vi "cm2nm_index_and_pair_fiducials.vi"(2 "CurrentSessionCollectionOfPoints":T1[](array[typedef]), 4 "ReferenceSessionCollectionOfPoints":T1[](array[typedef]), 5 "IndexCurrentSession_PairingList":i32[](array[numeric]), 6 "ReplacePairedFidName":bool, 7 "ReferenceSessionFiducialIndex":i32[](array[numeric]), 8 "CurrentSessionFiducialIndex":i32[](array[numeric]), 9 "IndexRefrenceSession_PairlingList":i32[](array[numeric])) -> (0 "CurrentSessionOut":T1[](array[typedef])=[{"MetaDataFile"=path "", "X"=-1.1, "Y"=0.0, "Z"=0.0, "Group"=0, "Rotation"=0.0, "Fiducial"=TRUE, "Magnification"=0.0, "Working_Distance"=0.0, "Notes"="", "Location Name/ID"="", "OtherRelatedDataFiles"=[], "Available"=FALSE}, {"MetaDataFile"=path "", "X"=0.0, "Y"=-1.0, "Z"=0.0, "Group"=0, "Rotation"=0.0, "Fiducial"=TRUE, "Magnification"=0.0, "Working_Distance"=0.0, "Notes"="", "Location Name/ID"="", "OtherRelatedDataFiles"=[], "Available"=FALSE}, {"MetaDataFile"=path "", "X"=0.0, "Y"=1.0, "Z"=0.0, "Group"=0, "Rotation"=0.0, "Fiducial"=TRUE, "Magnification"=0.0, "Working_Distance"=0.0, "Notes"="", "Location Name/ID"="", "OtherRelatedDataFiles"=[], "Available"=FALSE}, {"MetaDataFile"=path "", "X"=1.0, "Y"=0.0, "Z"=0.0, "Group"=0, "Rotation"=0.0, "Fiducial"=TRUE, "Magnification"=0.0, "Working_Distance"=0.0, "Notes"="", "Location Name/ID"="", "OtherRelatedDataFiles"=[], "Available"=FALSE}], 1 "PairedFiducialNames":T2(array[cluster]), 3 "PairedFiducials":T3(array[cluster]))   [LabVIEW 2011]
doc: "This Vi extracts the paired coordinates and names and puts into the format that the coordinate transform functions where created. Just book keeping."
uses:
  cm2nm_coordinate_information_v2.ctl
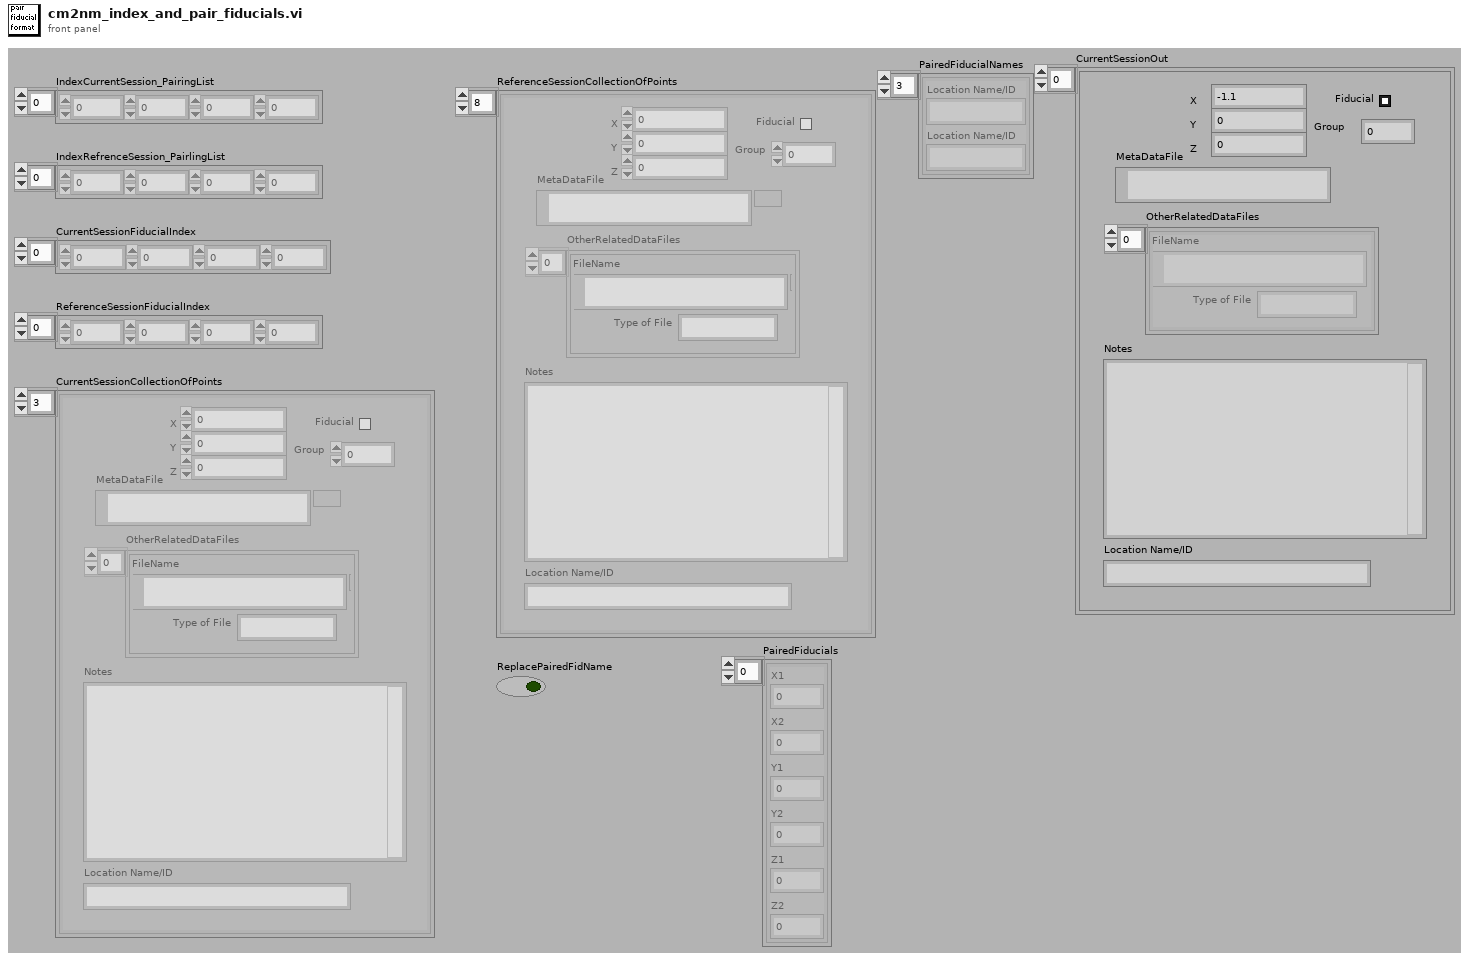
[diagram p1: front panel]
types:
  T1 = typedef "cm2nm_coordinate_information_v2.ctl" = cluster{"MetaDataFile":path, "X":dbl, "Y":dbl, "Z":dbl, "Group":i32, "Rotation":dbl[unit], "Fiducial":bool, "Magnification":dbl, "Working_Distance":dbl, "Notes":string, "Location Name/ID":string, "OtherRelatedDataFiles":cluster{"Type of File":string, "FileName":path}[], "Available":bool}
  T2 = cluster{"Location Name/ID":string, "Location Name/ID":string}[]
  T3 = cluster{"X1":dbl, "X2":dbl, "Y1":dbl, "Y2":dbl, "Z1":dbl, "Z2":dbl}[]
  T4 = cluster{"X1":dbl, "X2":dbl, "Y1":dbl, "Y2":dbl, "Z1":dbl, "Z2":dbl}
  T5 = cluster{"Location Name/ID":string, "Location Name/ID":string}
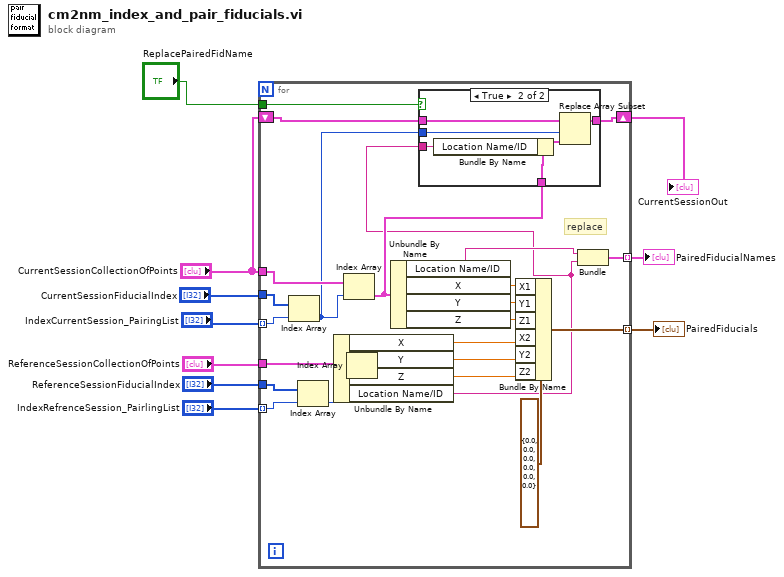
[diagram p0: block diagram]
diagram:
  n1 = for {
    tunnel: "IndexRefrenceSession_PairlingList" -> [w32] mode=indexing
    tunnel: "ReferenceSessionFiducialIndex" -> [w31]
    tunnel: "CurrentSessionFiducialIndex" -> [w33]
    tunnel: "IndexCurrentSession_PairingList" -> [w34] mode=indexing
    tunnel: "CurrentSessionCollectionOfPoints" -> [w17]
    tunnel: "ReferenceSessionCollectionOfPoints" -> [w29]
    tunnel: [w20] -> w10 mode=indexing
    tunnel: [w18] -> w4 mode=indexing
    shift-right: [w12] -> w2
    shift-left: "CurrentSessionCollectionOfPoints" -> [w15]
    tunnel: "ReplacePairedFidName" -> [w11]
    # "replace"
    n2 = Index Array(array=w33, index=w34) -> (element=w16:i32)
    n3 = Index Array(array=w31, index=w32) -> (element=w30:i32)
    n4 = Index Array(array=w17, index=w16) -> (element=w14:T1)
    n5 = Index Array(array=w29, index=w30) -> (element=w28:T1)
    n6 = Unbundle By Name(w28) -> ("X"=w24:dbl, "Y"=w23:dbl, "Z"=w22:dbl, "Location Name/ID"=w13:string)
    n7 = Unbundle By Name(w14) -> ("Location Name/ID"=w19:string, "X"=w27:dbl, "Y"=w26:dbl, "Z"=w25:dbl)
    n8 = case shown="True" w11 {
      tunnel: w16 -> [_ w41]
      tunnel: w15 -> [w35 w40]
      tunnel: w14 -> [_ w39]
      tunnel: w13 -> [_ w37]
      tunnel: [w35 w36] -> w12
      frame False {
      }
      frame True {
        n9 = Bundle By Name(cluster=w39, "Location Name/ID"=w37) -> (w38:T1)
        n10 = Replace Array Subset(array=w40, new element=w38, index=w41) -> (w36:T1[])
      }
    }
    n11 = Bundle By Name(cluster=T4 {"X1"=0.0, "X2"=0.0, "Y1"=0.0, "Y2"=0.0, "Z1"=0.0, "Z2"=0.0} ("Cluster"), "X1"=w27, "Y1"=w26, "Z1"=w25, "X2"=w24, "Y2"=w23, "Z2"=w22) -> (w20:T4)
    n12 = Bundle("Location Name/ID"=w19, "Location Name/ID"=w13) -> (w18:T5)  [unwired: 1 out]
  }
  "PairedFiducials" <- w10
  "PairedFiducialNames" <- w4
  "CurrentSessionOut" <- w2
